vi "Register gRPC Messages.vi"(8 "error in (no error)":errorcluster, 11 "gRPC ID":T1) -> (0 "error out":errorcluster, 3 "gRPC ID Out":T1)   [LabVIEW 2021, in "NI Measurement V2 Client.lvlib"]
uses:
  NI Measurement V2 Client.lvlib
  <vilib>/gRPC/LabVIEW gRPC Library/Shared/grpcId.ctl
  <vilib>/gRPC/LabVIEW gRPC Library/Server API/typeDefs/Message Metadata.ctl
  <vilib>/gRPC/LabVIEW gRPC Library/Server API/typeDefs/Message Element Metadata.ctl
  <vilib>/gRPC/LabVIEW gRPC Library/Server API/typeDefs/Message Element Type.ctl
  <vilib>/gRPC/LabVIEW gRPC Library/Server API/typeDefs/Enum Metadata.ctl
  <vilib>/gRPC/LabVIEW gRPC Library/grpc-lvsupport-release.lvlib
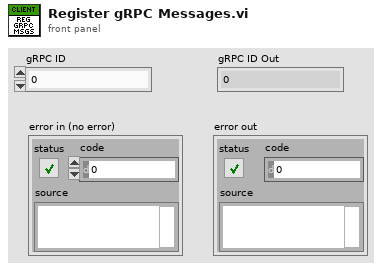
[diagram p1: front panel]
types:
  T1 = typedef "grpc-lvsupport-release.lvlib/grpcId.ctl" = u64
  T2 = typedef "grpc-lvsupport-release.lvlib/Enum Metadata.ctl" = cluster{"Version":i32, "Name":string, "Type Url":string, "Enum Values":string, "Allow Alias":bool}
  T3 = typedef "grpc-lvsupport-release.lvlib/Message Metadata.ctl" = cluster{"Version":i32, "Name":string, "Type Url":string, "Elements":T4[], "Has Oneof":bool}
  T4 = typedef "grpc-lvsupport-release.lvlib/Message Element Metadata.ctl" = cluster{"Field Name":string, "Embedded Message Name":string, "Protobuf Index":i32, "MessageElementType":T5, "Repeated":bool, "Is in Oneof":bool, "Oneof Container Name":string}
  T5 = typedef "grpc-lvsupport-release.lvlib/Message Element Type.ctl" = enum32{"Int32Value", "FloatValue", "DoubleValue", "BoolValue", "StringValue", "MessageValue", "Int64Value", "UInt32Value", "UInt64Value", "EnumValue", "Bytes", "Fixed64", "Fixed32", "SFixed64", "SFixed32", "SInt64", "SInt32"}
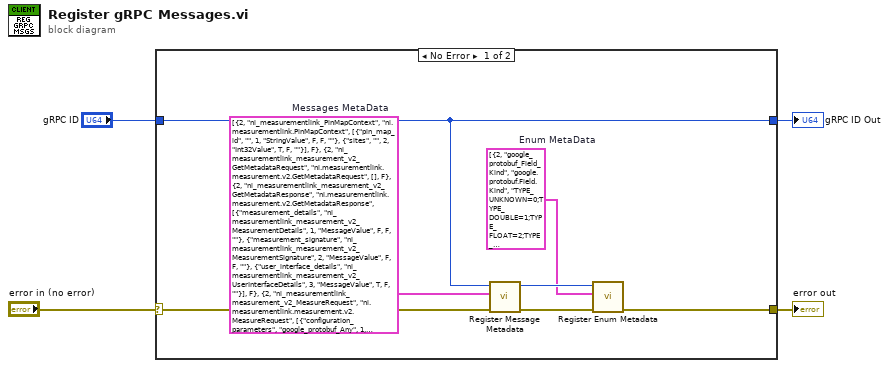
[diagram p0: block diagram]
diagram:
  n1 = case shown="No Error" "error in (no error)" {
    selector: "error in (no error)" -> [w10 w13]
    tunnel: [w9 w12] -> w1
    tunnel: [w6 w13] -> w4
    tunnel: "gRPC ID" -> [w9 w12]
    frame No Error {
      w5 = T2[] [{"Version"=2, "Name"="google_protobuf_Field_Kind", "Type Url"="google.protobuf.Field.Kind", "Enum Values"="TYPE_UNKNOWN=0;TYPE_DOUBLE=1;TYPE_FLOAT=2;TYPE_INT64=3;TYPE_UINT64=4;TYPE_INT32=5;TYPE_FIXED64=6;TYPE_FIXED32=7;TYPE_BOOL=8;TYPE_STRING=9;TYPE_GROUP=10;TYPE_MESSAGE=11;TYPE_BYTES=12;TYPE_UINT32=13;TYPE_ENUM=14;TYPE_SFIXED32=15;TYPE_SFIXED64=16;TYPE_SINT32=17;TYPE_SINT64=18", "Allow Alias"=FALSE}, {"Version"=2, "Name"="google_protobuf_Field_Cardinality", "Type Url"="google.protobuf.Field.Cardinality", "Enum Values"="CARDINALITY_UNKNOWN=0;CARDINALITY_OPTIONAL=1;CARDINALITY_REQUIRED=2;CARDINALITY_REPEATED=3", "Allow Alias"=FALSE}, {"Version"=2, "Name"="google_protobuf_Syntax", "Type Url"="google.protobuf.Syntax", "Enum Values"="SYNTAX_PROTO2=0;SYNTAX_PROTO3=1", "Allow Alias"=FALSE}]  # Enum MetaData
      w11 = T3[] [{"Version"=2, "Name"="ni_measurementlink_PinMapContext", "Type Url"="ni.measurementlink.PinMapContext", "Elements"=[{"Field Name"="pin_map_id", "Embedded Message Name"="", "Protobuf Index"=1, "MessageElementType"=enum."StringValue", "Repeated"=FALSE, "Is in Oneof"=FALSE, "Oneof Container Name"=""}, {"Field Name"="sites", "Embedded Message Name"="", "Protobuf Index"=2, "MessageElementType"=enum."Int32Value", "Repeated"=TRUE, "Is in Oneof"=FALSE, "Oneof Container Name"=""}], "Has Oneof"=FALSE}, {"Version"=2, "Name"="ni_measurementlink_measurement_v2_GetMetadataRequest", "Type Url"="ni.measurementlink.measurement.v2.GetMetadataRequest", "Elements"=[], "Has Oneof"=FALSE}, {"Version"=2, "Name"="ni_measurementlink_measurement_v2_GetMetadataResponse", "Type Url"="ni.measurementlink.measurement.v2.GetMetadataResponse", "Elements"=[{"Field Name"="measurement_details", "Embedded Message Name"="ni_measurementlink_measurement_v2_MeasurementDetails", "Protobuf Index"=1, "MessageElementType"=enum."MessageValue", "Repeated"=FALSE, "Is in Oneof"=FALSE, "Oneof Container Name"=""}, {"Field Name"="measurement_signature", "Embedded Message Name"="ni_measurementlink_measurement_v2_MeasurementSignature", "Protobuf Index"=2, "MessageElementType"=enum."MessageValue", "Repeated"=FALSE, "Is in Oneof"=FALSE, "Oneof Container Name"=""}, {"Field Name"="user_interface_details", "Embedded Message Name"="ni_measurementlink_measurement_v2_UserInterfaceDetails", "Protobuf Index"=3, "MessageElementType"=enum."MessageValue", "Repeated"=TRUE, "Is in Oneof"=FALSE, "Oneof Container Name"=""}], "Has Oneof"=FALSE}, {"Version"=2, "Name"="ni_measurementlink_measurement_v2_MeasureRequest", "Type Url"="ni.measurementlink.measurement.v2.MeasureRequest", "Elements"=[{"Field Name"="configuration_parameters", "Embedded Message Name"="google_protobuf_Any", "Protobuf Index"=1, "MessageElementType"=enum."MessageValue", "Repeated"=FALSE, "Is in Oneof"=FALSE, "Oneof Container Name"=""}, {"Field Name"="pin_map_context", "Embedded Message Name"="ni_measurementlink_PinMapContext", "Protobuf Index"=2, "MessageElementType"=enum."MessageValue", "Repeated"=FALSE, "Is in Oneof"=FALSE, "Oneof Container Name"=""}], "Has Oneof"=FALSE}, {"Version"=2, "Name"="ni_measurementlink_measurement_v2_MeasureResponse", "Type Url"="ni.measurementlink.measurement.v2.MeasureResponse", "Elements"=[{"Field Name"="outputs", "Embedded Message Name"="google_protobuf_Any", "Protobuf Index"=1, "MessageElementType"=enum."MessageValue", "Repeated"=FALSE, "Is in Oneof"=FALSE, "Oneof Container Name"=""}], "Has Oneof"=FALSE}, {"Version"=2, "Name"="ni_measurementlink_measurement_v2_MeasurementDetails", "Type Url"="ni.measurementlink.measurement.v2.MeasurementDetails", "Elements"=[{"Field Name"="display_name", "Embedded Message Name"="", "Protobuf Index"=1, "MessageElementType"=enum."StringValue", "Repeated"=FALSE, "Is in Oneof"=FALSE, "Oneof Container Name"=""}, {"Field Name"="version", "Embedded Message Name"="", "Protobuf Index"=2, "MessageElementType"=enum."StringValue", "Repeated"=FALSE, "Is in Oneof"=FALSE, "Oneof Container Name"=""}], "Has Oneof"=FALSE}, {"Version"=2, "Name"="ni_measurementlink_measurement_v2_MeasurementSignature", "Type Url"="ni.measurementlink.measurement.v2.MeasurementSignature", "Elements"=[{"Field Name"="configuration_parameters_message_type", "Embedded Message Name"="", "Protobuf Index"=1, "MessageElementType"=enum."StringValue", "Repeated"=FALSE, "Is in Oneof"=FALSE, "Oneof Container Name"=""}, {"Field Name"="configuration_parameters", "Embedded Message Name"="ni_measurementlink_measurement_v2_ConfigurationParameter", "Protobuf Index"=2, "MessageElementType"=enum."MessageValue", "Repeated"=TRUE, "Is in Oneof"=FALSE, "Oneof Container Name"=""}, {"Field Name"="configuration_defaults", "Embedded Message Name"="google_protobuf_Any", "Protobuf Index"=3, "MessageElementType"=enum."MessageValue", "Repeated"=FALSE, "Is in Oneof"=FALSE, "Oneof Container Name"=""}, {"Field Name"="outputs_message_type", "Embedded Message Name"="", "Protobuf Index"=4, "MessageElementType"=enum."StringValue", "Repeated"=FALSE, "Is in Oneof"=FALSE, "Oneof Container Name"=""}, {"Field Name"="outputs", "Embedded Message Name"="ni_measurementlink_measurement_v2_Output", "Protobuf Index"=5, "MessageElementType"=enum."MessageValue", "Repeated"=TRUE, "Is in Oneof"=FALSE, "Oneof Container Name"=""}], "Has Oneof"=FALSE}, {"Version"=2, "Name"="ni_measurementlink_measurement_v2_UserInterfaceDetails", "Type Url"="ni.measurementlink.measurement.v2.UserInterfaceDetails", "Elements"=[{"Field Name"="file_url", "Embedded Message Name"="", "Protobuf Index"=1, "MessageElementType"=enum."StringValue", "Repeated"=FALSE, "Is in Oneof"=FALSE, "Oneof Container Name"=""}], "Has Oneof"=FALSE}, {"Version"=2, "Name"="ni_measurementlink_measurement_v2_ConfigurationParameter", "Type Url"="ni.measurementlink.measurement.v2.ConfigurationParameter", "Elements"=[{"Field Name"="field_number", "Embedded Message Name"="", "Protobuf Index"=1, "MessageElementType"=enum."Int32Value", "Repeated"=FALSE, "Is in Oneof"=FALSE, "Oneof Container Name"=""}, {"Field Name"="type", "Embedded Message Name"="google_protobuf_Field_Kind", "Protobuf Index"=2, "MessageElementType"=enum."EnumValue", "Repeated"=FALSE, "Is in Oneof"=FALSE, "Oneof Container Name"=""}, {"Field Name"="name", "Embedded Message Name"="", "Protobuf Index"=3, "MessageElementType"=enum."StringValue", "Repeated"=FALSE, "Is in Oneof"=FALSE, "Oneof Container Name"=""}, {"Field Name"="repeated", "Embedded Message Name"="", "Protobuf Index"=4, "MessageElementType"=enum."BoolValue", "Repeated"=FALSE, "Is in Oneof"=FALSE, "Oneof Container Name"=""}, {"Field Name"="annotations", "Embedded Message Name"="ni_measurementlink_measurement_v2_ConfigurationParameter_AnnotationsEntry", "Protobuf Index"=5, "MessageElementType"=enum."MessageValue", "Repeated"=TRUE, "Is in Oneof"=FALSE, "Oneof Container Name"=""}, {"Field Name"="message_type", "Embedded Message Name"="", "Protobuf Index"=6, "MessageElementType"=enum."StringValue", "Repeated"=FALSE, "Is in Oneof"=FALSE, "Oneof Container Name"=""}], "Has Oneof"=FALSE}, {"Version"=2, "Name"="ni_measurementlink_measurement_v2_Output", "Type Url"="ni.measurementlink.measurement.v2.Output", "Elements"=[{"Field Name"="field_number", "Embedded Message Name"="", "Protobuf Index"=1, "MessageElementType"=enum."Int32Value", "Repeated"=FALSE, "Is in Oneof"=FALSE, "Oneof Container Name"=""}, {"Field Name"="type", "Embedded Message Name"="google_protobuf_Field_Kind", "Protobuf Index"=2, "MessageElementType"=enum."EnumValue", "Repeated"=FALSE, "Is in Oneof"=FALSE, "Oneof Container Name"=""}, {"Field Name"="name", "Embedded Message Name"="", "Protobuf Index"=3, "MessageElementType"=enum."StringValue", "Repeated"=FALSE, "Is in Oneof"=FALSE, "Oneof Container Name"=""}, {"Field Name"="repeated", "Embedded Message Name"="", "Protobuf Index"=4, "MessageElementType"=enum."BoolValue", "Repeated"=FALSE, "Is in Oneof"=FALSE, "Oneof Container Name"=""}, {"Field Name"="annotations", "Embedded Message Name"="ni_measurementlink_measurement_v2_Output_AnnotationsEntry", "Protobuf Index"=5, "MessageElementType"=enum."MessageValue", "Repeated"=TRUE, "Is in Oneof"=FALSE, "Oneof Container Name"=""}, {"Field Name"="message_type", "Embedded Message Name"="", "Protobuf Index"=6, "MessageElementType"=enum."StringValue", "Repeated"=FALSE, "Is in Oneof"=FALSE, "Oneof Container Name"=""}], "Has Oneof"=FALSE}, {"Version"=2, "Name"="ni_measurementlink_measurement_v2_ConfigurationParameter_AnnotationsEntry", "Type Url"="ni.measurementlink.measurement.v2.ConfigurationParameter.AnnotationsEntry", "Elements"=[{"Field Name"="key", "Embedded Message Name"="", "Protobuf Index"=1, "MessageElementType"=enum."StringValue", "Repeated"=FALSE, "Is in Oneof"=FALSE, "Oneof Container Name"=""}, {"Field Name"="value", "Embedded Message Name"="", "Protobuf Index"=2, "MessageElementType"=enum."StringValue", "Repeated"=FALSE, "Is in Oneof"=FALSE, "Oneof Container Name"=""}], "Has Oneof"=FALSE}, {"Version"=2, "Name"="google_protobuf_Any", "Type Url"="google.protobuf.Any", "Elements"=[{"Field Name"="type_url", "Embedded Message Name"="", "Protobuf Index"=1, "MessageElementType"=enum."StringValue", "Repeated"=FALSE, "Is in Oneof"=FALSE, "Oneof Container Name"=""}, {"Field Name"="value", "Embedded Message Name"="", "Protobuf Index"=2, "MessageElementType"=enum."Bytes", "Repeated"=FALSE, "Is in Oneof"=FALSE, "Oneof Container Name"=""}], "Has Oneof"=FALSE}, {"Version"=2, "Name"="google_protobuf_SourceContext", "Type Url"="google.protobuf.SourceContext", "Elements"=[{"Field Name"="file_name", "Embedded Message Name"="", "Protobuf Index"=1, "MessageElementType"=enum."StringValue", "Repeated"=FALSE, "Is in Oneof"=FALSE, "Oneof Container Name"=""}], "Has Oneof"=FALSE}, {"Version"=2, "Name"="google_protobuf_Type", "Type Url"="google.protobuf.Type", "Elements"=[{"Field Name"="name", "Embedded Message Name"="", "Protobuf Index"=1, "MessageElementType"=enum."StringValue", "Repeated"=FALSE, "Is in Oneof"=FALSE, "Oneof Container Name"=""}, {"Field Name"="fields", "Embedded Message Name"="google_protobuf_Field", "Protobuf Index"=2, "MessageElementType"=enum."MessageValue", "Repeated"=TRUE, "Is in Oneof"=FALSE, "Oneof Container Name"=""}, {"Field Name"="oneofs", "Embedded Message Name"="", "Protobuf Index"=3, "MessageElementType"=enum."StringValue", "Repeated"=TRUE, "Is in Oneof"=FALSE, "Oneof Container Name"=""}, {"Field Name"="options", "Embedded Message Name"="google_protobuf_Option", "Protobuf Index"=4, "MessageElementType"=enum."MessageValue", "Repeated"=TRUE, "Is in Oneof"=FALSE, "Oneof Container Name"=""}, {"Field Name"="source_context", "Embedded Message Name"="google_protobuf_SourceContext", "Protobuf Index"=5, "MessageElementType"=enum."MessageValue", "Repeated"=FALSE, "Is in Oneof"=FALSE, "Oneof Container Name"=""}, {"Field Name"="syntax", "Embedded Message Name"="google_protobuf_Syntax", "Protobuf Index"=6, "MessageElementType"=enum."EnumValue", "Repeated"=FALSE, "Is in Oneof"=FALSE, "Oneof Container Name"=""}], "Has Oneof"=FALSE}, {"Version"=2, "Name"="google_protobuf_Field", "Type Url"="google.protobuf.Field", "Elements"=[{"Field Name"="kind", "Embedded Message Name"="google_protobuf_Field_Kind", "Protobuf Index"=1, "MessageElementType"=enum."EnumValue", "Repeated"=FALSE, "Is in Oneof"=FALSE, "Oneof Container Name"=""}, {"Field Name"="cardinality", "Embedded Message Name"="google_protobuf_Field_Cardinality", "Protobuf Index"=2, "MessageElementType"=enum."EnumValue", "Repeated"=FALSE, "Is in Oneof"=FALSE, "Oneof Container Name"=""}, {"Field Name"="number", "Embedded Message Name"="", "Protobuf Index"=3, "MessageElementType"=enum."Int32Value", "Repeated"=FALSE, "Is in Oneof"=FALSE, "Oneof Container Name"=""}, {"Field Name"="name", "Embedded Message Name"="", "Protobuf Index"=4, "MessageElementType"=enum."StringValue", "Repeated"=FALSE, "Is in Oneof"=FALSE, "Oneof Container Name"=""}, {"Field Name"="type_url", "Embedded Message Name"="", "Protobuf Index"=6, "MessageElementType"=enum."StringValue", "Repeated"=FALSE, "Is in Oneof"=FALSE, "Oneof Container Name"=""}, {"Field Name"="oneof_index", "Embedded Message Name"="", "Protobuf Index"=7, "MessageElementType"=enum."Int32Value", "Repeated"=FALSE, "Is in Oneof"=FALSE, "Oneof Container Name"=""}, {"Field Name"="packed", "Embedded Message Name"="", "Protobuf Index"=8, "MessageElementType"=enum."BoolValue", "Repeated"=FALSE, "Is in Oneof"=FALSE, "Oneof Container Name"=""}, {"Field Name"="options", "Embedded Message Name"="google_protobuf_Option", "Protobuf Index"=9, "MessageElementType"=enum."MessageValue", "Repeated"=TRUE, "Is in Oneof"=FALSE, "Oneof Container Name"=""}, {"Field Name"="json_name", "Embedded Message Name"="", "Protobuf Index"=10, "MessageElementType"=enum."StringValue", "Repeated"=FALSE, "Is in Oneof"=FALSE, "Oneof Container Name"=""}, {"Field Name"="default_value", "Embedded Message Name"="", "Protobuf Index"=11, "MessageElementType"=enum."StringValue", "Repeated"=FALSE, "Is in Oneof"=FALSE, "Oneof Container Name"=""}], "Has Oneof"=FALSE}, {"Version"=2, "Name"="google_protobuf_Enum", "Type Url"="google.protobuf.Enum", "Elements"=[{"Field Name"="name", "Embedded Message Name"="", "Protobuf Index"=1, "MessageElementType"=enum."StringValue", "Repeated"=FALSE, "Is in Oneof"=FALSE, "Oneof Container Name"=""}, {"Field Name"="enumvalue", "Embedded Message Name"="google_protobuf_EnumValue", "Protobuf Index"=2, "MessageElementType"=enum."MessageValue", "Repeated"=TRUE, "Is in Oneof"=FALSE, "Oneof Container Name"=""}, {"Field Name"="options", "Embedded Message Name"="google_protobuf_Option", "Protobuf Index"=3, "MessageElementType"=enum."MessageValue", "Repeated"=TRUE, "Is in Oneof"=FALSE, "Oneof Container Name"=""}, {"Field Name"="source_context", "Embedded Message Name"="google_protobuf_SourceContext", "Protobuf Index"=4, "MessageElementType"=enum."MessageValue", "Repeated"=FALSE, "Is in Oneof"=FALSE, "Oneof Container Name"=""}, {"Field Name"="syntax", "Embedded Message Name"="google_protobuf_Syntax", "Protobuf Index"=5, "MessageElementType"=enum."EnumValue", "Repeated"=FALSE, "Is in Oneof"=FALSE, "Oneof Container Name"=""}], "Has Oneof"=FALSE}, {"Version"=2, "Name"="google_protobuf_EnumValue", "Type Url"="google.protobuf.EnumValue", "Elements"=[{"Field Name"="name", "Embedded Message Name"="", "Protobuf Index"=1, "MessageElementType"=enum."StringValue", "Repeated"=FALSE, "Is in Oneof"=FALSE, "Oneof Container Name"=""}, {"Field Name"="number", "Embedded Message Name"="", "Protobuf Index"=2, "MessageElementType"=enum."Int32Value", "Repeated"=FALSE, "Is in Oneof"=FALSE, "Oneof Container Name"=""}, {"Field Name"="options", "Embedded Message Name"="google_protobuf_Option", "Protobuf Index"=3, "MessageElementType"=enum."MessageValue", "Repeated"=TRUE, "Is in Oneof"=FALSE, "Oneof Container Name"=""}], "Has Oneof"=FALSE}, {"Version"=2, "Name"="google_protobuf_Option", "Type Url"="google.protobuf.Option", "Elements"=[{"Field Name"="name", "Embedded Message Name"="", "Protobuf Index"=1, "MessageElementType"=enum."StringValue", "Repeated"=FALSE, "Is in Oneof"=FALSE, "Oneof Container Name"=""}, {"Field Name"="value", "Embedded Message Name"="google_protobuf_Any", "Protobuf Index"=2, "MessageElementType"=enum."MessageValue", "Repeated"=FALSE, "Is in Oneof"=FALSE, "Oneof Container Name"=""}], "Has Oneof"=FALSE}, {"Version"=2, "Name"="ni_measurementlink_measurement_v2_Output_AnnotationsEntry", "Type Url"="ni.measurementlink.measurement.v2.Output.AnnotationsEntry", "Elements"=[{"Field Name"="key", "Embedded Message Name"="", "Protobuf Index"=1, "MessageElementType"=enum."StringValue", "Repeated"=FALSE, "Is in Oneof"=FALSE, "Oneof Container Name"=""}, {"Field Name"="value", "Embedded Message Name"="", "Protobuf Index"=2, "MessageElementType"=enum."StringValue", "Repeated"=FALSE, "Is in Oneof"=FALSE, "Oneof Container Name"=""}], "Has Oneof"=FALSE}]  # Messages MetaData
      n2 = call <vilib>:"Register Message Metadata.vi"("error in"=w10, "Messages"=w11, "gRPCid in"=w9) -> ("error out"=w7:errorcluster, "gRPCid out"=w8:T1)  [unwired: 7 in]
      n3 = call <vilib>:"Register Enum Metadata.vi"("error in"=w7, "Enum Metadata"=w5, "gRPCid in"=w8) -> ("error out"=w6:errorcluster)  [unwired: 7 in, 1 out]
    }
    frame Error {
    }
  }
  "error out" <- w4
  "gRPC ID Out" <- w1
